vi "NIDAQmx Logic.vi"(8 "error in (no error)":errorcluster, 9 "channel":string, 10 "Session Factory in":refnum<class "Session Factory.lvclass">, 11 "Measurement Configuration":T2) -> (0 "error out":errorcluster, 3 "Measurement Results":T1)   [LabVIEW 2021, in "NIDAQmxMeasurement.lvlib"]
doc: "This example demonstrates how to measure a finite single frequency sample. It uses implicit timing, \nwhich means that a sample is acquired for every period of your input signal. The Set Channel Property \n(CI Frequency Input Terminal and CI Frequency Measurement) helps specify the input terminal of \nthe signal to measure and the duration for measuring the signal frequency.\n\nFor more information, see the DAQmx \nexample: <examples>\\DAQmx\\Counter Input\\Counter - Read Pulse Width and Frequency (Finite).vi"
uses:
  NIDAQmxMeasurement.lvlib
  Measurement Configuration.ctl
  Measurement Results.ctl
  Source/Sessions/niDAQmx/Session Factory/Session Factory.lvclass
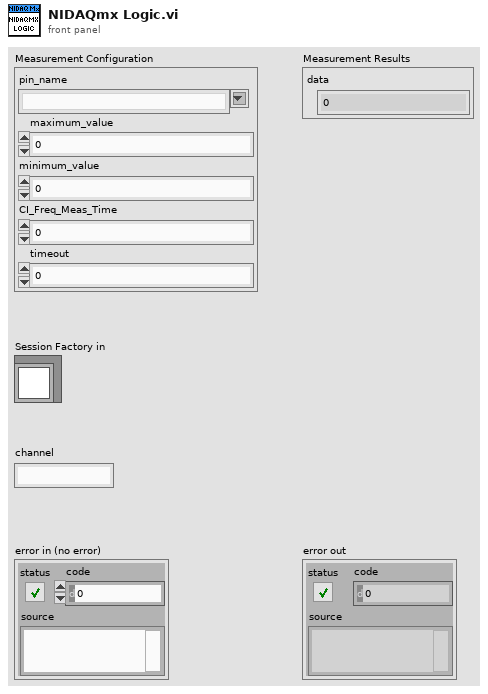
[diagram p1: front panel]
types:
  T1 = typedef "NIDAQmxMeasurement.lvlib/Measurement Results.ctl" = cluster{"data":dbl}
  T2 = typedef "NIDAQmxMeasurement.lvlib/Measurement Configuration.ctl" = cluster{"pin_name":string, "maximum_value":dbl, "minimum_value":dbl, "CI_Freq_Meas_Time":dbl, "timeout":dbl}
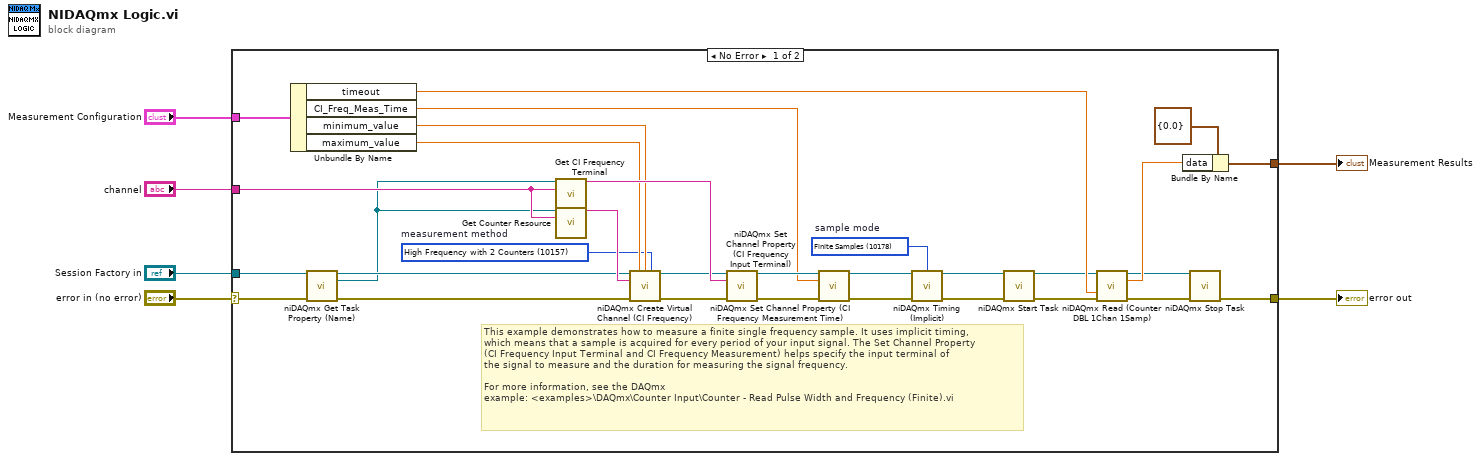
[diagram p0: block diagram]
diagram:
  n1 = case shown="No Error" "error in (no error)" {
    selector: "error in (no error)" -> [w11 w38]
    tunnel: "Measurement Configuration" -> [w37 _]
    tunnel: [w36 _] -> w5
    tunnel: [w24 w38] -> w4
    tunnel: "Session Factory in" -> [w8 _]
    tunnel: "channel" -> [w12 _]
    frame No Error {
      w25 = 10157 items=["Low Frequency with 1 Counter"=10105, "High Frequency with 2 Counters"=10157, "Large Range with 2 Counters"=10205, "Dynamic Averaging"=16065]  # measurement method
      w28 = 10178 items=["Finite Samples"=10178, "Continuous Samples"=10123, "Hardware Timed Single Point"=12522]  # sample mode
      # "This example demonstrates how to measure a finite single frequency sample. It uses implicit timing, \nwhich means that a sample is acquired for every period of your input signal. The Set Channel Property \n(CI Frequency Input Terminal and CI Frequency Measurement) helps specify the input terminal of \nthe signal to measure and the duration for measuring the signal frequency.\n\nFor more information, see the DAQmx \nexample: <examples>\\DAQmx\\Counter Input\\Counter - Read Pulse Width and Frequency (Finite).vi"
      n2 = Unbundle By Name(w37) -> ("timeout"=w33:dbl, "CI_Freq_Meas_Time"=w13:dbl, "minimum_value"=w29:dbl, "maximum_value"=w30:dbl)
      n3 = call "niDAQmx Get Task Property (Name).vi"("task in"=w8, "error in"=w11) -> ("task out"=w9:refnum<class "Session Factory.lvclass">, "Name"=w7:refnum<k21>, "error out"=w10:errorcluster)  [unwired: 11 in]
      n4 = call "Get CI Frequency Terminal.vi"("Task Name"=w7, "channel"=w12) -> ("CI.Freq.Term"=w32:tag)  [unwired: 13 in]
      n5 = call "Get Counter Resource.vi"("Task Name"=w7, "channel"=w12) -> ("counter"=w31:tag)  [unwired: 13 in]
      n6 = call "niDAQmx Create Virtual Channel (CI Frequency).vi"("task in"=w9, "maximum value"=w30, "minimum value"=w29, "measurement method"=w25, "counter"=w31, "error in"=w10) -> ("task out"=w19:refnum<class "Session Factory.lvclass">, "error out"=w18:errorcluster)  [unwired: 8 in]
      n7 = call "niDAQmx Set Channel Property (CI Frequency Input Terminal).vi"("task in"=w19, "CI.Freq.Term"=w32, "error in"=w18) -> ("task out"=w15:refnum<class "Session Factory.lvclass">, "error out"=w17:errorcluster)  [unwired: 11 in]
      n8 = call "niDAQmx Set Channel Property (CI Frequency Measurement Time).vi"("task in"=w15, "CI.Freq.MeasTime"=w13, "error in"=w17) -> ("task out"=w14:refnum<class "Session Factory.lvclass">, "error out"=w16:errorcluster)  [unwired: 11 in]
      n9 = call "niDAQmx Timing (Implicit).vi"("task in"=w14, "sample mode"=w28, "error in"=w16) -> ("task out"=w27:refnum<class "Session Factory.lvclass">, "error out"=w26:errorcluster)  [unwired: 11 in]
      n10 = call "niDAQmx Start Task.vi"("task in"=w27, "error in"=w26) -> ("task out"=w22:refnum<class "Session Factory.lvclass">, "error out"=w20:errorcluster)  [unwired: 12 in]
      n11 = call "niDAQmx Read (Counter DBL 1Chan 1Samp).vi"("task in"=w22, "timeout"=w33, "error in"=w20) -> ("task out"=w23:refnum<class "Session Factory.lvclass">, "data"=w35:dbl, "error out"=w21:errorcluster)  [unwired: 10 in]
      n12 = Bundle By Name(cluster=T1 {"data"=0.0} ("Measurement Results"), "data"=w35) -> (w36:T1)
      n13 = call "niDAQmx Stop Task.vi"("task in"=w23, "error in"=w21) -> ("error out"=w24:errorcluster)  [unwired: 12 in, 1 out]
    }
    frame Error {
    }
  }
  "Measurement Results" <- w5
  "error out" <- w4
